vi "Read power_.vi"(8 "error in (no error)":errorcluster, 11 "Update Meerstetter Ctl Val in":refnum<class "Update Meerstetter Ctl Val.lvclass">) -> (0 "error out":errorcluster, 2 "power?":bool, 3 "Update Meerstetter Ctl Val out":refnum<class "Update Meerstetter Ctl Val.lvclass">)   [LabVIEW 2014, in "Controller.lvlib" / "Update Meerstetter Ctl Val.lvclass"]
uses:
  Update Meerstetter Ctl Val.lvclass
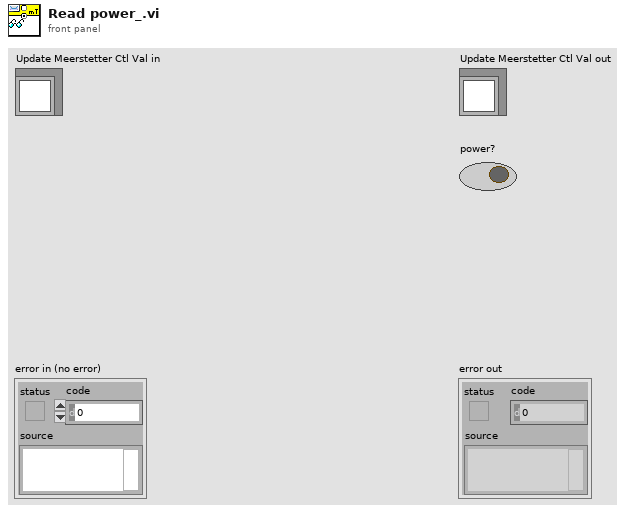
[diagram p1: front panel]
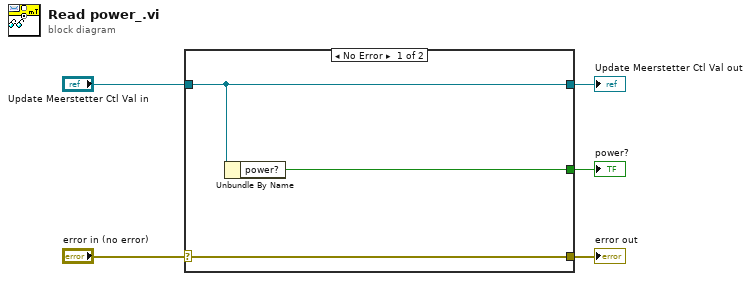
[diagram p0: block diagram]
diagram:
  n1 = case shown="No Error" "error in (no error)" {
    selector: "error in (no error)" -> [w8 w9]
    tunnel: [w8 w9] -> w4
    tunnel: [w7 w10] -> w2
    tunnel: "Update Meerstetter Ctl Val in" -> [w7 w10]
    tunnel: [w6 _] -> w1
    frame No Error {
      n2 = Unbundle By Name(w7) -> ("power?"=w6:bool)
    }
    frame Error {
    }
  }
  "error out" <- w4
  "Update Meerstetter Ctl Val out" <- w2
  "power?" <- w1
